vi "Texture.vi"(8 "error in (no error)":errorcluster, 11 "Image":T1) -> (0 "error out":errorcluster, 3 "New Texture Refnum":refnum<vi>)   [LabVIEW 2020, in "NI_3D Picture Control.lvlib"]
doc: "Creates a new texture from an image and applies the texture to the surface of an object in the 3D scene."
uses:
  <vilib>/picture/3D Picture Control/NI_3D Picture Control.lvlib
  <vilib>/picture/picture.llb/imagedata.ctl
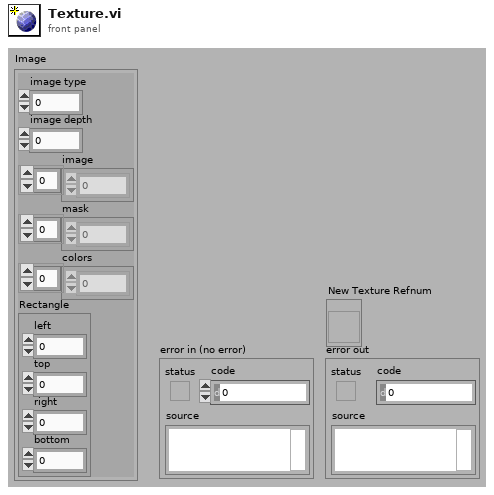
[diagram p1: front panel]
types:
  T1 = typedef "imagedata.ctl" = cluster{"image type":i32, "image depth":i32, "image":u8[], "mask":u8[], "colors":u32[], "Rectangle":cluster{"left":i16, "top":i16, "right":i16, "bottom":i16}}
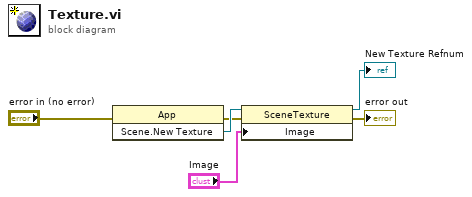
[diagram p0: block diagram]
diagram:
  n1 = invoke class="App" method="Scene.New Texture"(error in="error in (no error)") -> (error out=w1:errorcluster, "Scene.New Texture"=w4:refnum<vi>)  [unwired: 2 in, 1 out]
  n2 = property class="SceneTexture"(reference=w4, error in=w1, "Image"="Image") -> (reference out=→"New Texture Refnum":refnum<vi>, error out=→"error out":errorcluster)
